vi "ConnectDevice.vi"(8 "error in (no error)":errorcluster caption="错误输入（无错误）", 10 "DeviceInd":u32, 11 "type":u16(ring)=2 items=["USB-CAN"=2, "USB-CAN2.0"=3]) -> (0 "error out":errorcluster caption="错误输出", 3 "success":bool)   [LabVIEW 2011]
uses:
  data/ControlCAN.dll
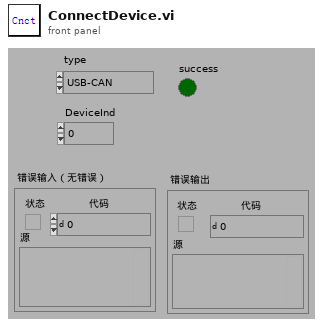
[diagram p1: front panel]
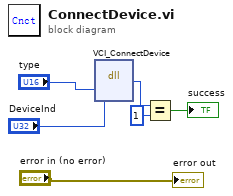
[diagram p0: block diagram]
diagram:
  n1 = dll-call lib="PTH1Nabs D\t董海成\t上位机2.进行中USB-CAN TooldataControlCAN.dll" fn="VCI_ConnectDevice"("DeviceType"="type", "DeviceInd"="DeviceInd") -> ("返回类型"=w6:u32)  [unwired: 5 in, 2 out]
  n2 = Equal?(x=w6, y=u32 1) -> (x = y?=→"success":bool)
  "error out" <- "error in (no error)"
